vi "Wristband main - Pinch Leap based.vi"() -> ()   [LabVIEW 2014]
uses:
  Typedef/sensor_data.ctl
  Typedef/flexext_data.ctl
  Typedef/pinch_data.ctl
  SubVIs/Save Blocks - 2D.vi
  <vilib>/MakerHub/LINX/Public/Peripherals/Analog/Analog Read N Chans.vi
  <vilib>/MakerHub/LINX/LMH-LINX.lvlib
panel:
  out "Spread":u8
  in  "Spread  Button 2":bool
  out "Pinch cluster":T1
  in  "Clear Plot":bool
  in  "Acquire":bool
  in  "Tacq":u32=50 caption="Acquisition Interval" min=50 max=10000 step=50 format="%.0fms"
  in  "N pts":i32=500
  in  "Session name":string="Session 0"
  in  "Save to path":path=path "C:/Users/Andrea/Desktop/Progetto Canada/Dati"
  out "Leap \nConnected?":bool=TRUE caption="Leap Motion"
  in  "Arduino Port":refnum<visa-resource-name>="COM20"
  out "Status":bool=TRUE caption="Arduino"
  out "Sensor Chart":T2(graph)={"Sensor  Chan 0"=1.2451171875, "Sensor Chan 2"=1.2353515625, "Sensor Chan 4"=1.240234375, "Sensor Chan 5"=1.2255859375}
  out "Grab Strength":u8
  out "Flexext cluster":T3
  out "Sensor Data":T4={"Sensor  Chan 0"=1.25, "Sensor Chan 1"=1.240234375, "Sensor Chan 2"=1.2353515625, "Sensor Chan 3"=1.240234375, "Sensor Chan 4"=1.2353515625, "Sensor Chan 5"=1.220703125}
  in  "Exit":bool=TRUE
  out "Event Chart":T5(graph)
  # "Connection panel"
  # "Acquisition panel"
  # "Save settings"
  # "Connection status"
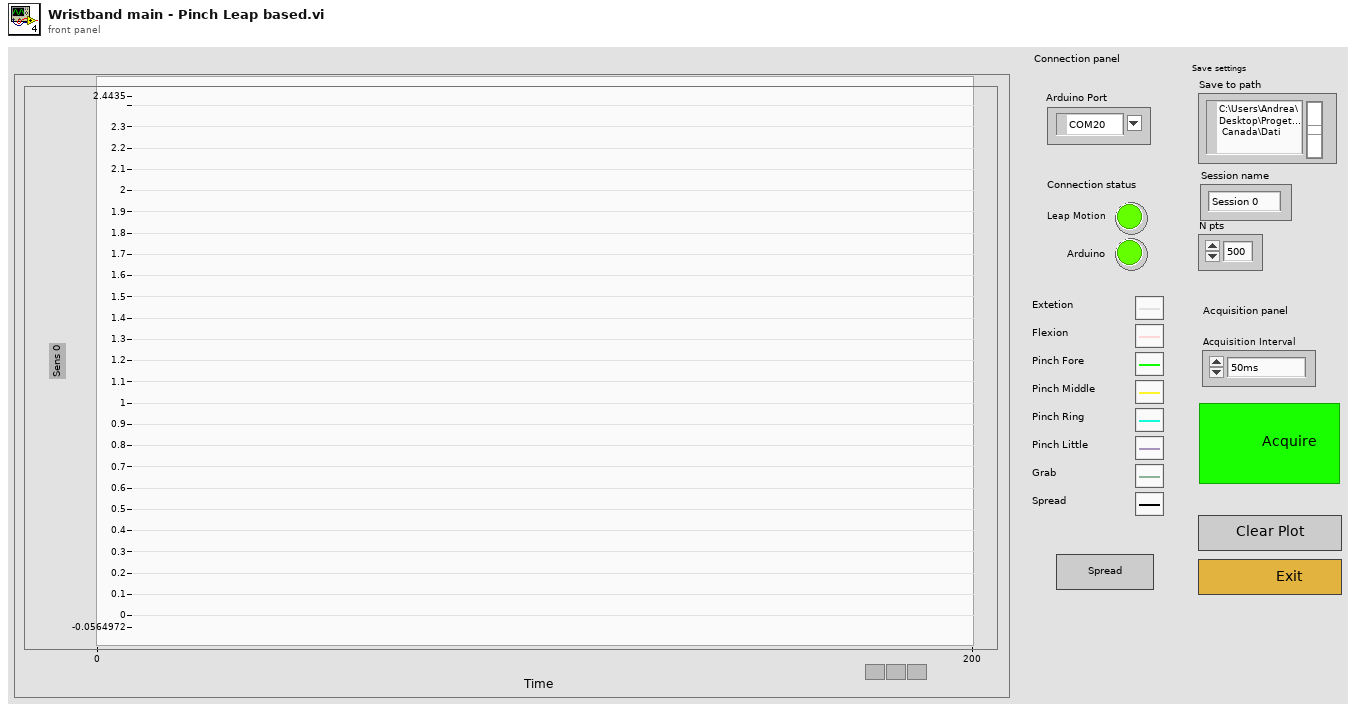
[diagram p1: front panel]
types:
  T1 = typedef "pinch_data.ctl" = cluster{"Indice":u8, "Medio":u8, "Anulare":u8, "Mignolo":u8}
  T2 = cluster{"Sensor  Chan 0":dbl, "Sensor Chan 2":dbl, "Sensor Chan 4":dbl, "Sensor Chan 5":dbl}
  T3 = typedef "flexext_data.ctl" = cluster{"Estensione":u8, "Flessione":u8}
  T4 = typedef "Sensor_data.ctl" = cluster{"Sensor  Chan 0":dbl, "Sensor Chan 1":dbl, "Sensor Chan 2":dbl, "Sensor Chan 3":dbl, "Sensor Chan 4":dbl, "Sensor Chan 5":dbl}
  T5 = cluster{"Estensione":u8, "Flessione":u8, "Pollice":u8, "Indice":u8, "Medio":u8, "Anulare":u8, "Mignolo":u8, "Grab Strength":u8}
  T6 = typedef "LMH-LINX.lvlib/LINX Ref.ctl" = cluster{"Platform":T7, "Interface":T8, "LINX Device Config":T9}
  T7 = typedef "LMH-LINX.lvlib/Platform.ctl" = enum16{"LINX", "myRIO"}
  T8 = typedef "LMH-LINX.lvlib/Interface.ctl" = enum16{"Serial", "TCP"}
  T9 = typedef "LMH-LINX.lvlib/Device.lvlib/LINX Device Config.ctl" = cluster{"Interface":T8, "COM Port":refnum<visa-resource-name>, "TCP Configuration":T10, "Device Family":u8, "Device ID":u8, "Device Name":string, "TCP Ref":refnum<k5>, "Channels":T11}
  T10 = typedef "LMH-LINX.lvlib/Device.lvlib/TCP Config.ctl" = cluster{"IP Address":string, "Port":u16}
  T11 = typedef "LMH-LINX.lvlib/Channels.ctl" = cluster{"DI":u8[], "DO":u8[], "AI":u8[], "AO":u8[], "PWM":u8[], "QE":u8[], "UART":u8[], "I2C 2":u8[], "SPI":u8[], "CAN":u8[], "Servo":u8[], "AI Ref (V)":dbl, "AO Ref (V)":dbl, "AO Resolution (Bits)":u8}
  T12 = typedef "Leap Handle.ctl" = cluster{"LeapCSharp":refnum<k24>}
  T13 = cluster{"Sensor  Chan 0":dbl, "Sensor Chan 2":dbl, "Sensor Chan 4":dbl, "Sensor Chan 5":dbl}[]
  T14 = cluster{"Estensione":u8, "Flessione":u8, "Pollice":u8, "Indice":u8, "Medio":u8, "Anulare":u8, "Mignolo":u8, "Grab Strength":u8}[]
  T15 = cluster{"Sensor  Chan 0":dbl, "Sensor Chan 1":dbl, "Sensor Chan 2":dbl, "Sensor Chan 3":dbl}
  T16 = cluster{"Estensione":u8, "Flessione":u8, "Indice":u8, "Medio":u8, "Anulare":u8, "Mignolo":u8, "Grab Strength":u8, "Spread":u8}
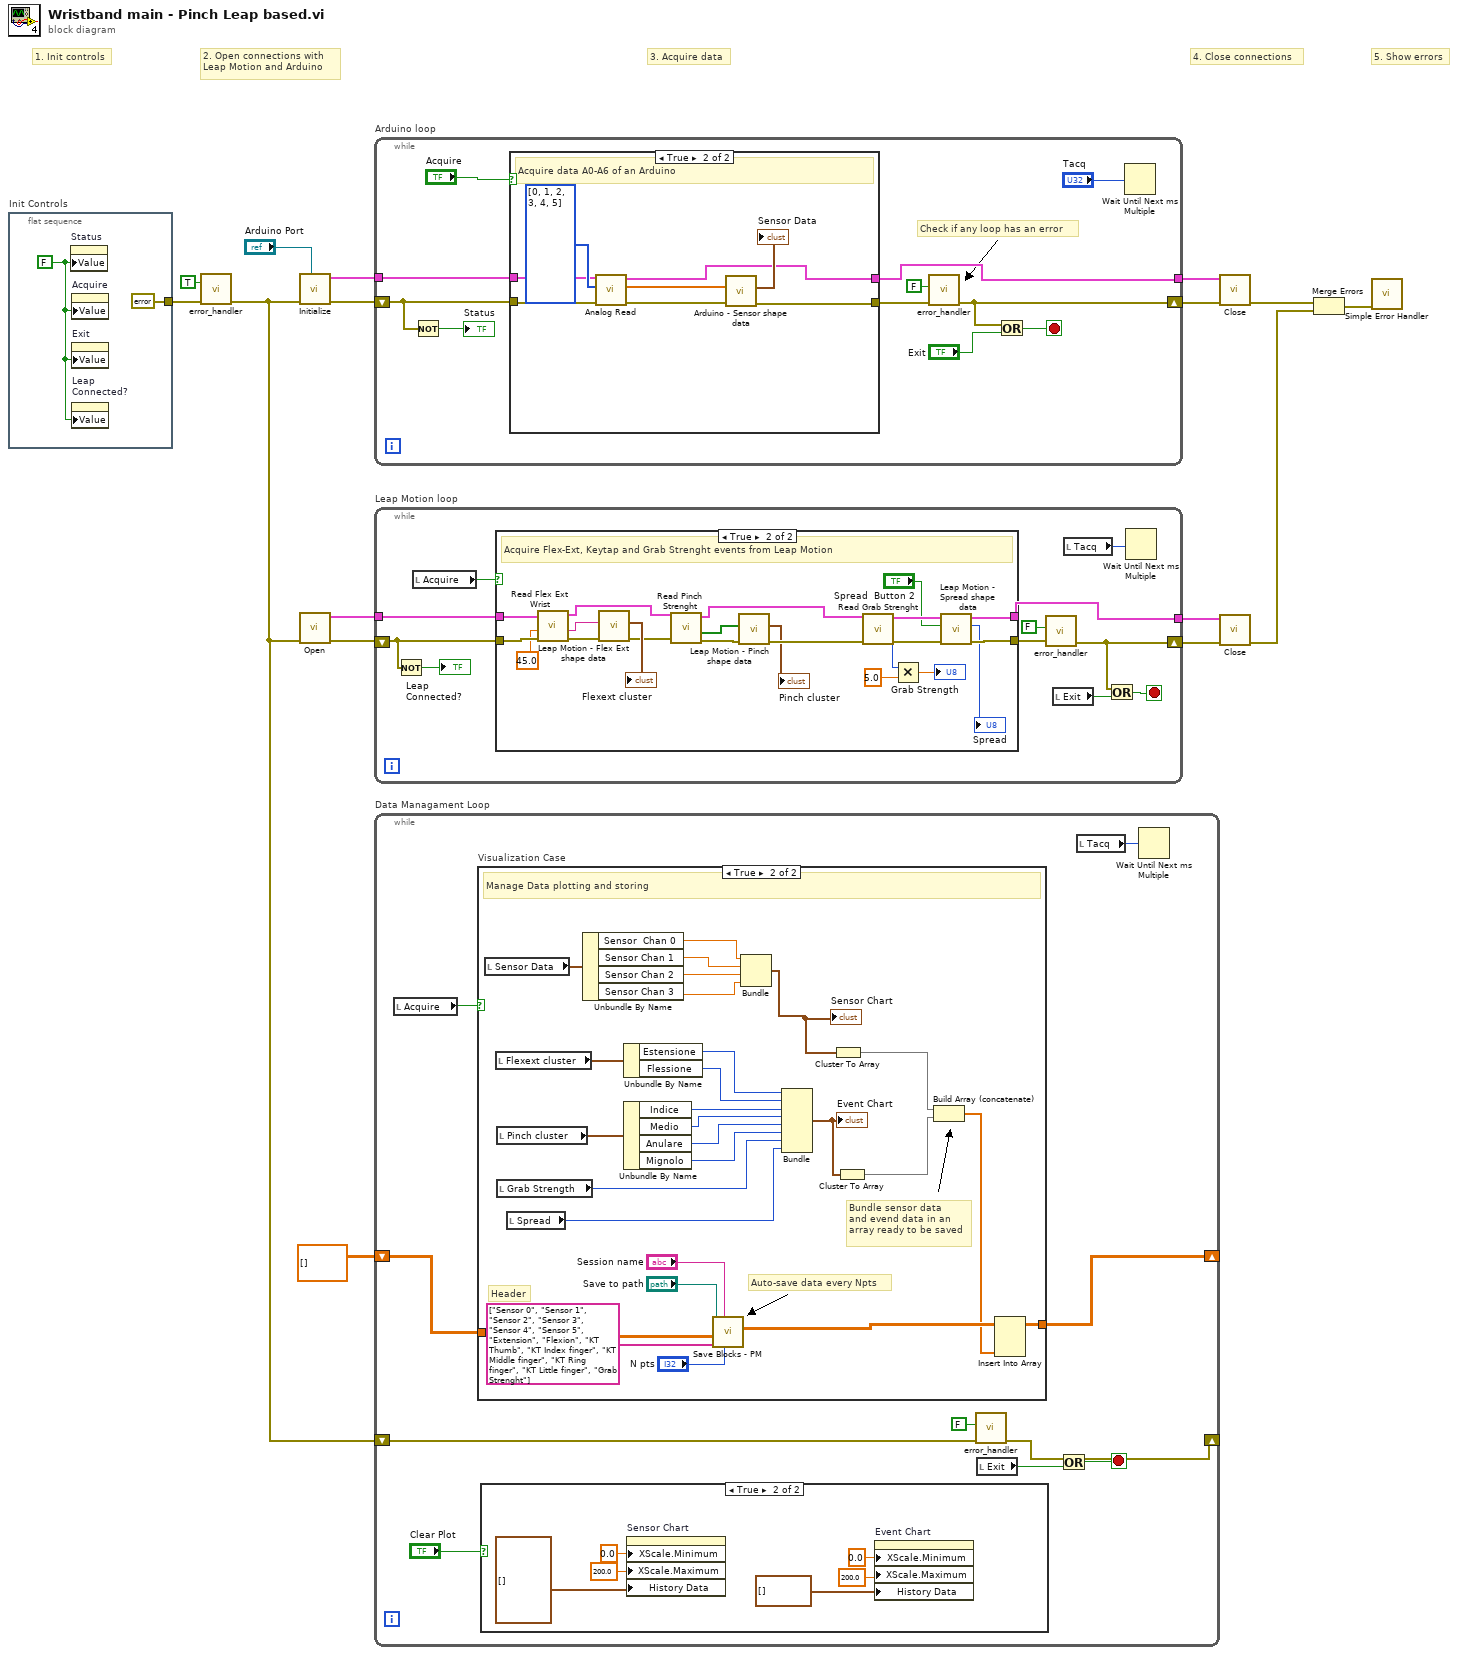
[diagram p0: block diagram]
diagram:
  # "5. Show errors"
  # "4. Close connections"
  # "3. Acquire data"
  # "2. Open connections with\nLeap Motion and Arduino"
  # "1. Init controls"
  n1 = flat-sequence "Init Controls" {
    tunnel: [errorcluster {"status"=FALSE, "code"=0, "source"=""} ("Error In")] -> w7
    frame #0 {
      w17 = FALSE ("Status")
      n2 = property on="Status" class="Bool (strict)"("Value"=w17) -> ()  [unwired: 2 in, 2 out]
      n3 = property on="Acquire" class="Bool (strict)"("Value"=w17) -> ()  [unwired: 2 in, 2 out]
      n4 = property on="Exit" class="Bool (strict)"("Value"=w17) -> ()  [unwired: 2 in, 2 out]
      n5 = property on="Leap \nConnected?" class="Bool (strict)"("Value"=w17) -> ()  [unwired: 2 in, 2 out]
    }
  }
  n6 = call "error_handler.vi"("Error In"=w7, "Reset"=TRUE) -> ("Error Out"=w6:errorcluster)  [unwired: 9 in]
  n7 = call <vilib>:"Initialize.vi"("Serial Port"="Arduino Port", "Error In"=w6) -> ("Error Out"=w15:errorcluster, "LINX Ref"=w16:T6)  [unwired: 7 in, 1 out]
  n8 = call "Open.vi"("Error In"=w6) -> ("Error Out"=w10:errorcluster, "Leap Handle"=w11:T12)  [unwired: 9 in]
  n9 = while "Arduino loop" {
    tunnel: w16 -> [w28]
    tunnel: [w20] -> w12
    shift-right: [w21] -> w13
    shift-left: w15 -> [w24]
    stop <- w26 stop-if-true
    # "Check if any loop has an error"
    n10 = Not(x=w24) -> (.not. x?=→"Status":bool)
    n11 = case shown="True" "Acquire" {
      tunnel: w28 -> [w30 w37]
      tunnel: w24 -> [w31 w39]
      tunnel: [w30 w32] -> w20
      tunnel: [w31 w35] -> w22
      frame False {
        # "Idle"
      }
      frame True {
        # "Acquire data A0-A6 of an Arduino"
        n12 = call-poly <vilib>:"Analog Read.vi"("Error In"=w39, "AI Channel(s)"=u8[] [0, 1, 2, 3, 4, 5], "LINX Resource"=w37) -> ("Error Out"=w36:errorcluster, "Voltages"=w34:dbl[], "LINX Resource"=w32:T6)  [unwired: 5 in, 1 out]
        n13 = call "Arduino - Sensor shape data.vi"("Error In"=w36, "Sensor Data in"=w34) -> ("Error Out"=w35:errorcluster, "Sensor Data Out"=→"Sensor Data":T4)  [unwired: 8 in]
      }
    }
    n14 = call "error_handler.vi"("Error In"=w22, "Reset"=FALSE) -> ("Error Out"=w21:errorcluster)  [unwired: 9 in]
    n15 = Or(x=w21, y="Exit") -> (x .or. y?=w26:bool)
    n16 = Wait Until Next ms Multiple(millisecond multiple="Tacq") -> ()  [unwired: 1 out]
  }
  n17 = while "Leap Motion loop" {
    tunnel: w11 -> [w48]
    tunnel: [w42] -> w9
    shift-right: [w44] -> w8
    shift-left: w10 -> [w41]
    stop <- w49 stop-if-true
    n18 = Not(x=w41) -> (.not. x?=→"Leap \nConnected?":bool)
    n19 = local read "Acquire"() -> (w46:bool)
    n20 = case shown="True" w46 {
      tunnel: w48 -> [w52 w73]
      tunnel: w41 -> [w51 w72]
      tunnel: [w52 w67] -> w42
      tunnel: [w51 w55] -> w45
      frame False {
        # "Idle"
      }
      frame True {
        # "Acquire Flex-Ext, Keytap and Grab Strenght events from Leap Motion"
        n21 = call "Read Flex Ext Wrist.vi"("Error In"=w72, "Flex Extension threshold"=sgl 45.0, "Leap Handle In"=w73) -> ("Error Out"=w70:errorcluster, "Wrist Flextion/Extension"=w69:string, "Leap Handle Out"=w62:T12)  [unwired: 4 in]
        n22 = call "Leap Motion - Flex Ext shape data.vi"("Error In"=w70, "Event In"=w69) -> ("Error Out"=w63:errorcluster, "Flexext cluster"=→"Flexext cluster":T3)  [unwired: 8 in]
        n23 = call "Read Pinch Strenght.vi"("Error In"=w63, "Leap Handle In"=w62) -> ("Error Out"=w59:errorcluster, "Finger pinch"=w60:bool[], "Leap Handle Out"=w61:T12)  [unwired: 6 in, 1 out]
        n24 = call "Leap Motion - Pinch shape data.vi"("Error In"=w59, "Pinch"=w60) -> ("Error Out"=w58:errorcluster, "Pinch cluster"=→"Pinch cluster":T1)  [unwired: 8 in]
        n25 = call "Read Grab Strenght.vi"("Error In"=w58, "Leap Handle In"=w61) -> ("Error Out"=w56:errorcluster, "Numeric Palm State"=w64:i32, "Leap Handle Out"=w67:T12)  [unwired: 5 in, 2 out]
        n26 = Multiply(x=w64, y=sgl 5.0) -> (x*y=→"Grab Strength":sgl)
        n27 = call "Leap Motion - Spread shape data.vi"("Error In"=w56, "Spread  Button 2"="Spread  Button 2") -> ("Error Out"=w55:errorcluster, "Spread"=→"Spread":u8)  [unwired: 8 in]
      }
    }
    n28 = call "error_handler.vi"("Error In"=w45, "Reset"=FALSE) -> ("Error Out"=w44:errorcluster)  [unwired: 9 in]
    n29 = local read "Exit"() -> (w50:bool)
    n30 = local read "Tacq"() -> (w47:u32)
    n31 = Or(x=w44, y=w50) -> (x .or. y?=w49:bool)
    n32 = Wait Until Next ms Multiple(millisecond multiple=w47) -> ()  [unwired: 1 out]
  }
  n33 = while "Data Managament Loop" {
    shift-right: [w78] -> _
    shift-left: w6 -> [w79]
    shift-right: [w77] -> _
    shift-left: dbl[][] [] -> [w76]
    stop <- w80 stop-if-true
    n34 = local read "Acquire"() -> (w83:bool)
    n35 = case "Visualization Case" shown="True" w83 {
      tunnel: [w90 w109] -> w77
      tunnel: w76 -> [w90 w107]
      frame False {
        # "Idle"
      }
      frame True {
        # "Header"
        # "Auto-save data every Npts"
        # "Bundle sensor data\nand evend data in an\narray ready to be saved"
        # "Manage Data plotting and storing"
        n36 = local read "Sensor Data"() -> (w105:T4)
        n37 = local read "Flexext cluster"() -> (w117:T3)
        n38 = local read "Pinch cluster"() -> (w99:T1)
        n39 = local read "Grab Strength"() -> (w94:u8)
        n40 = local read "Spread"() -> (w93:u8)
        n41 = Unbundle By Name(w105) -> ("Sensor  Chan 0"=w104:dbl, "Sensor Chan 1"=w103:dbl, "Sensor Chan 2"=w102:dbl, "Sensor Chan 3"=w101:dbl)
        n42 = Unbundle By Name(w117) -> ("Estensione"=w116:u8, "Flessione"=w115:u8)
        n43 = Unbundle By Name(w99) -> ("Indice"=w98:u8, "Medio"=w97:u8, "Anulare"=w96:u8, "Mignolo"=w95:u8)
        n44 = call-poly "Save Blocks - PM.vi"("N pts"="N pts", "Session name"="Session name", "2D Data In"=w107, "Column headers"=string[] ["Sensor 0", "Sensor 1", "Sensor 2", "Sensor 3", "Sensor 4", "Sensor 5", "Extension", "Flexion", "KT Thumb", "KT Index finger", "KT Middle finger", "KT Ring finger", "KT Little finger", "Grab Strenght"], "Save to path"="Save to path") -> ("2D Data Out"=w113:dbl[][])  [unwired: 5 in, 1 out]
        n45 = Bundle("Sensor  Chan 0"=w104, "Sensor Chan 1"=w103, "Sensor Chan 2"=w102, "Sensor Chan 3"=w101) -> (w100:T15)  [unwired: 1 in]
        "Sensor Chart" <- w100
        n46 = Bundle("Estensione"=w116, "Flessione"=w115, "Indice"=w98, "Medio"=w97, "Anulare"=w96, "Mignolo"=w95, "Grab Strength"=w94, "Spread"=w93) -> (w92:T16)  [unwired: 1 in]
        "Event Chart" <- w92
        n47 = Cluster To Array(cluster=w100) -> (array=w114:dbl[])
        n48 = Cluster To Array(cluster=w92) -> (array=w91:u8[])
        n49 = Build Array (concatenate)(w114, w91) -> (w108:dbl[])
        n50 = Insert Into Array(array=w113, new element=w108) -> (w109:dbl[][])  [unwired: 2 in]
      }
    }
    n51 = case shown="True" "Clear Plot" {
      frame False {
      }
      frame True {
        n52 = property on="Sensor Chart" class="WFChart (strict)"("XScale.Minimum"=0.0 ("X Scale.Range:Minimum"), "XScale.Maximum"=200.0 ("X Scale.Range:Maximum"), "History Data"=T13 []) -> ()  [unwired: 2 in, 2 out]
        n53 = property on="Event Chart" class="WFChart (strict)"("XScale.Minimum"=0.0 ("X Scale.Range:Minimum"), "XScale.Maximum"=200.0 ("X Scale.Range:Maximum"), "History Data"=T14 []) -> ()  [unwired: 2 in, 2 out]
      }
    }
    n54 = call "error_handler.vi"("Error In"=w79, "Reset"=FALSE) -> ("Error Out"=w78:errorcluster)  [unwired: 9 in]
    n55 = local read "Exit"() -> (w81:bool)
    n56 = Or(x=w78, y=w81) -> (x .or. y?=w80:bool)
    n57 = local read "Tacq"() -> (w75:u32)
    n58 = Wait Until Next ms Multiple(millisecond multiple=w75) -> ()  [unwired: 1 out]
  }
  n59 = call <vilib>:"Close.vi"("Error In"=w13, "LINX Resource"=w12) -> ("Error Out"=w3:errorcluster)  [unwired: 8 in, 1 out]
  n60 = call <vilib>:"Close.vi"("Error In"=w8, "Leap Handle"=w9) -> ("Error Out"=w2:errorcluster)  [unwired: 9 in]
  n61 = Merge Errors(w3, w2) -> (w4:errorcluster)
  n62 = call <vilib>:"Simple Error Handler.vi"("error in (no error)"=w4) -> ()  [unwired: 4 in, 5 out]
